vi "Simulated VeriStand Engine.PCL.Stop.vi"(8 "error in (no error)":errorcluster, 11 "Simulated VeriStand Engine in":refnum<class "Simulated VeriStand Engine.lvclass">) -> (0 "error out":errorcluster, 2 "stop":bool, 3 "Simulated VeriStand Engine out":refnum<class "Simulated VeriStand Engine.lvclass">)   [LabVIEW 2016, in "Simulated VeriStand Engine.lvclass"]
uses:
  Simulated VeriStand Engine.lvclass
  Source/Submodules/Memory/Source/Classes/Internal/Memory.Pointer.Internal.lvclass
  C:/Git/SourceTree/DSF/Source/Submodules/Memory/Source/Classes/Pointer/Memory.Pointer.lvclass
  Source/Submodules/Memory/Source/Classes/Pointer/Memory.Pointer.lvclass/Memory.Pointer.ctl
  Source/Submodules/Memory/Source/Classes/Pointer/Memory.Pointer.Read.Safe.0D.Bool.vi
  Source/Submodules/Memory/Source/Classes/Pointer/Memory.Pointer.Read.Unsafe.0D.Bool.vi
  Source/Submodules/Memory/Source/Classes/Pointer/Memory.Pointer.Parameter Check.Null Pointer.vi
  Source/Submodules/Memory/Source/Classes/Pointer/Memory.Pointer.Parameter Check.Subset.vi
  Source/Submodules/Memory/Source/Classes/Pointer/Memory.Pointer.Get Address.vi
  Source/Submodules/Memory/Source/Classes/Pointer/Memory.Pointer.Errors.vi
  Source/Submodules/Memory/Source/Classes/Pointer/Memory.Pointer.Errors.Null Pointer.vi
  Source/Submodules/Memory/Source/Classes/Pointer/Memory.Pointer.Errors.Out of Bounds.vi
  Source/Submodules/Memory/Source/Classes/Pointer/Memory.Pointer.Get Size.vi
  Source/Submodules/Memory/Source/Classes/Pointer/Memory.Pointer.Errors.Create Error.vi
  Source/Submodules/Memory/Source/Submodules/SEH/Source/VIs/Static Error Handling.Source Buffer.Write.String.vi
  Source/Submodules/Memory/Source/Classes/Pointer/Memory.Pointer.Errors.Write Pointer Size.vi
  Source/Submodules/Memory/Source/Submodules/SEH/Source/VIs/Static Error Handling.Source Buffer.Write.Numeric.Scalar.Base10.vi
  Source/Submodules/Memory/Source/Submodules/SEH/Source/VIs/Static Error Handling.Source Buffer.Write.Numeric.Scalar.Base10 (U64).vi
  Source/Submodules/Memory/Source/Submodules/SEH/Source/VIs/Static Error Handling.Error Cluster Constant.vi
  Source/Submodules/Memory/Source/Submodules/SEH/Source/VIs/Static Error Handling.Error Cluster Constant (256B).vi
  Source/Submodules/Memory/Source/Submodules/SEH/Source/VIs/Static Error Handling.Parameters.Status.Set.vi
  Source/Submodules/Memory/Source/Submodules/SEH/Source/VIs/Static Error Handling.Parameters.Code.Set.vi
  Source/Submodules/Memory/Source/Submodules/SEH/Source/VIs/Static Error Handling.Parameters.VI Source.Set.vi
  Source/Submodules/Memory/Source/Constants/Memory.Constants.vi
  Source/Submodules/Memory/Source/Constants/Memory.Constants.Library Name.vi
  Source/Submodules/Memory/Source/Classes/Pointer/Memory.Pointer.Errors.Get Info.vi
  Source/Submodules/Memory/Source/Classes/Pointer/Memory.Pointer.lvclass
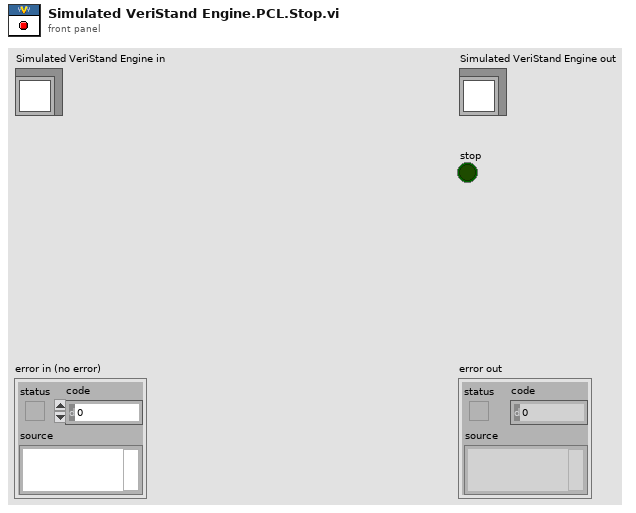
[diagram p1: front panel]
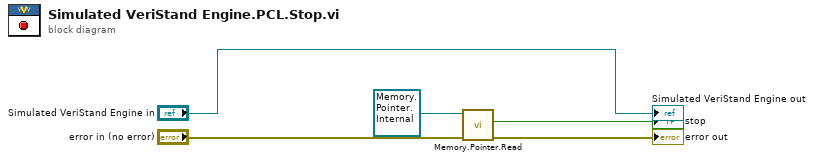
[diagram p0: block diagram]
diagram:
  n1 = call-poly "Memory.Pointer.Read.vi"("error in (no error)"="error in (no error)", "pointer in"=refnum<class "Memory.Pointer.Internal.lvclass"> refnum) -> ("error out"=→"error out":errorcluster, "value out"=→"stop":bool)  [unwired: 6 in, 2 out]
  "Simulated VeriStand Engine out" <- "Simulated VeriStand Engine in"
